vi "run_timeout.vi"() -> ()   [LabVIEW 2020]
panel:
  out "output":dbl
  in  "input":dbl=1.1 caption="x"
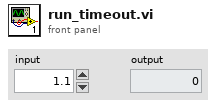
[diagram p1: front panel]
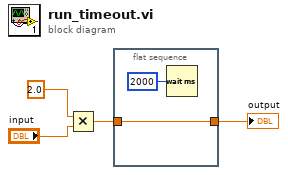
[diagram p0: block diagram]
diagram:
  n1 = Multiply(x=2.0, y="input") -> (x*y=w2:dbl)
  n2 = flat-sequence {
    tunnel: w2 -> [w5]
    tunnel: [w5] -> w1
    frame #0 {
      n3 = Wait (ms)(milliseconds to wait=u32 2000) -> ()  [unwired: 1 out]
    }
  }
  "output" <- w1
